vi "Constructor.vi"(11 "Sample Rate":i32) -> (3 "Sinusoidal Fit out":refnum<class "Sinusoidal Fit.lvclass">)   [LabVIEW 2016, in "Sinusoidal Fit.lvclass"]
uses:
  Sinusoidal Fit.lvclass
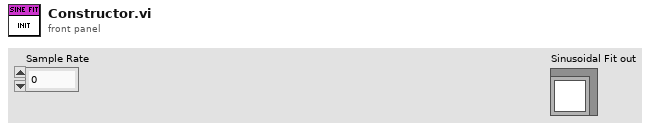
[diagram p1: front panel]
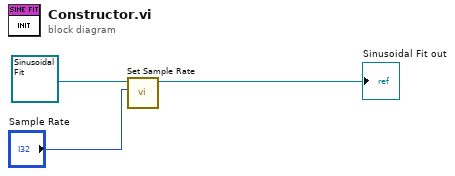
[diagram p0: block diagram]
diagram:
  n1 = call-dynamic "Set Sample Rate.vi"("Sample Rate"="Sample Rate", "Abstract Fit in"=refnum<class "Sinusoidal Fit.lvclass"> refnum ("Sinusoidal Fit.lvclass")) -> ("Abstract Fit out"=→"Sinusoidal Fit out":refnum<class "Sinusoidal Fit.lvclass">)  [unwired: 8 in, 1 out]
